vi "CDW_SpecPage.vi"(10 "Spec Page Interface":T2, 11 "MetaDataObj in":refnum<class "MetaDataObj.lvclass">) -> (3 "MetaDataObj out":refnum<class "MetaDataObj.lvclass">)   [LabVIEW 2015, in "NIVS_CDW_MetaDataObj.lvclass"]
uses:
  NIVS_CDW_MetaDataObj.lvclass
  <resource>/dialog/NewProjectWizard/Spec Page Interface.ctl
  <resource>/dialog/NewProjectWizard/MetaDataObj/MetaDataObj.lvclass
  <vilib>/Utility/sysdir.llb/System Directory Type.ctl
  TypDef/CD Wizard - Execution Mode.ctl
  NIVS_CDW_MetaDataObj.lvclass/NIVS_CDW_MetaDataObj.ctl
  <resource>/dialog/NewProjectWizard/MetaDataObj/MetaDataObj.lvclass/MetaDataObj.ctl
  TypDef/CD Wizard - Extra Page Name and GUID.ctl
  <resource>/dialog/NewProjectWizard/MetaDataObj/Accessors/Write Project Root.vi
  <resource>/dialog/NewProjectWizard/MetaDataObj/Accessors/Write Project Name.vi
panel:
  in  "Custom Device Execution Mode":T1(ring)=enum."Inline HW Interface"
  in  "Custom Device Name":string
  in  "Custom Device Path":path
  in  "Maximum Custom Device Instances":u32=1 min=1 max=2474 step=1
  in  "Insert Custom Device in submenu":bool
  in  "Parent Menu Name":string
  in  "Custom Device Extra Page Names":string[](array[string])
  # "Advanced Options"
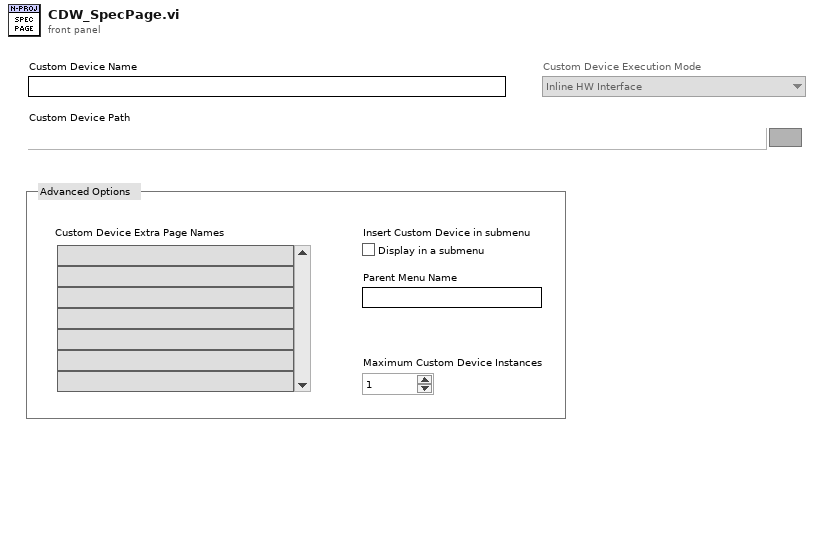
[diagram p1: front panel]
types:
  T1 = enum16{"Asynchronous", "Inline HW Interface", "Inline Model Interface", "Inline Timing and Sync", "Asynchronous Timing and Sync"}
  T2 = typedef "Spec Page Interface.ctl" = cluster{"\"Tab Forward To\" Refnum":refnum<vi>, "\"Tab Backward To\" Refnum":refnum<vi>, "Errors":refnum<user-event>, "Quit":refnum<user-event>}
  T3 = typedef "CD Wizard - Execution Mode.ctl" = enum16{"Asynchronous", "Inline HW Interface", "Inline Model Interface", "Inline Timing and Sync", "Asynchronous Timing and Sync"}
  T4 = typedef "System Directory Type.ctl" = i32
  T5 = enum8{"Enabled", "Disabled", "Disabled and Grayed Out"}
  T6 = cluster{"Insert CD in submenu":bool, "Parent Menu Name":string}
  T7 = typedef "CD Wizard - Extra Page Name and GUID.ctl" = cluster{"Page Name":string, "Page GUID":string}
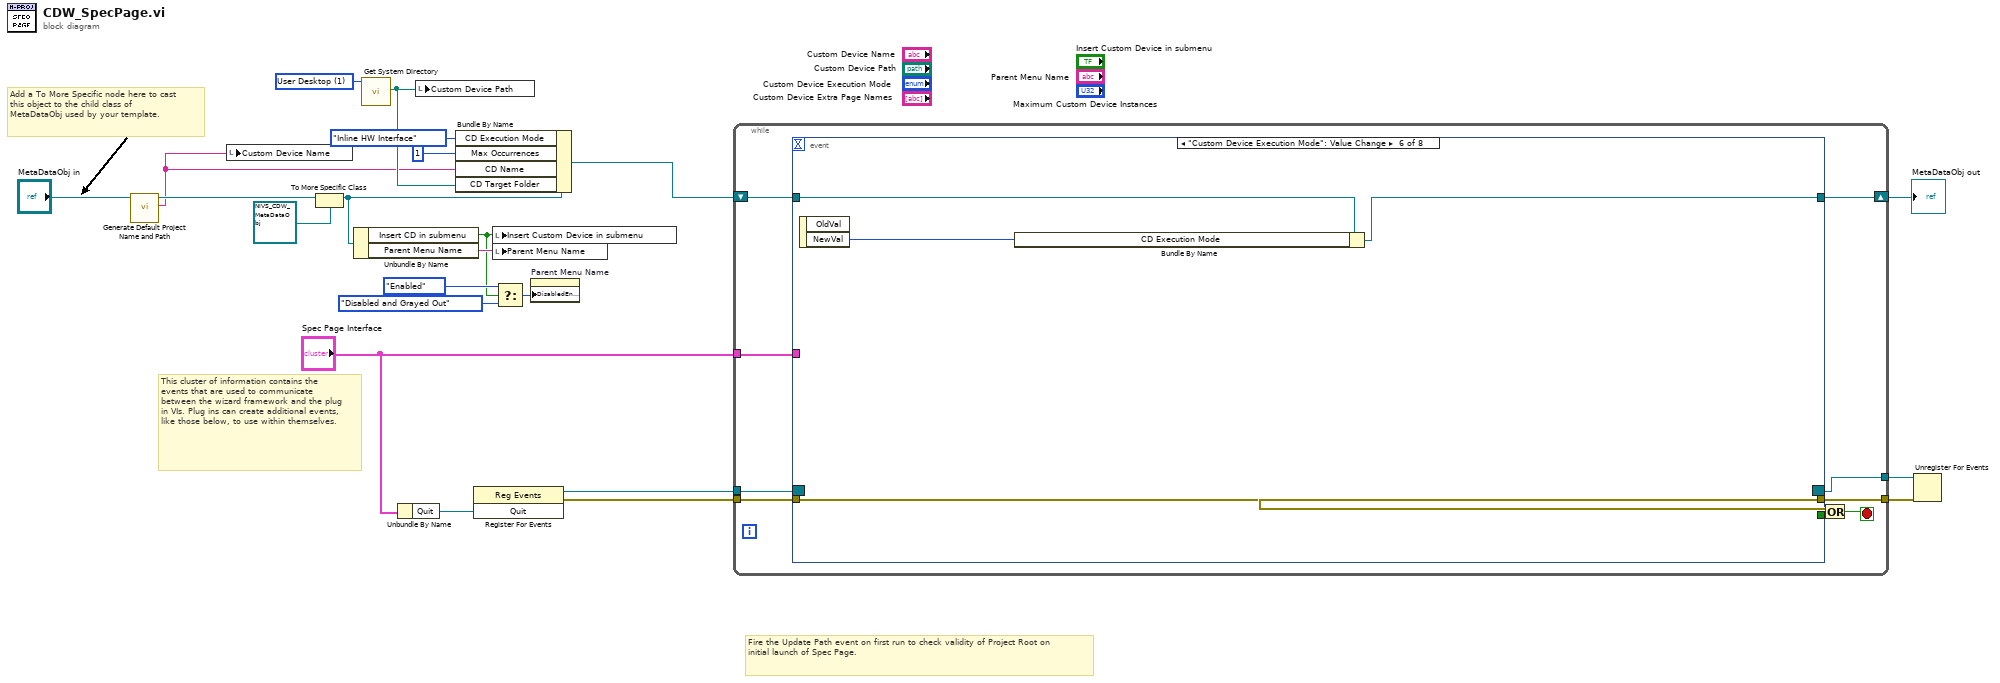
[diagram p0: block diagram]
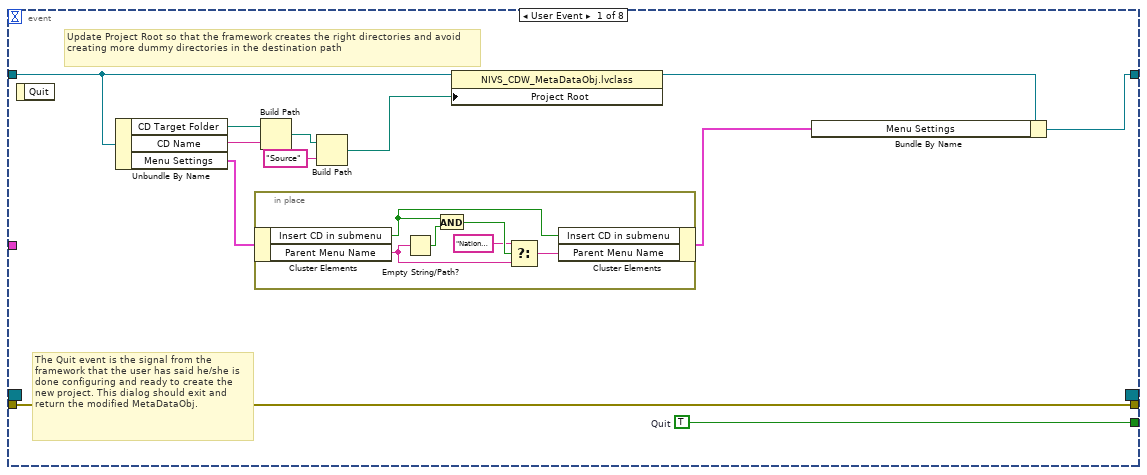
[diagram p2: hidden frame]
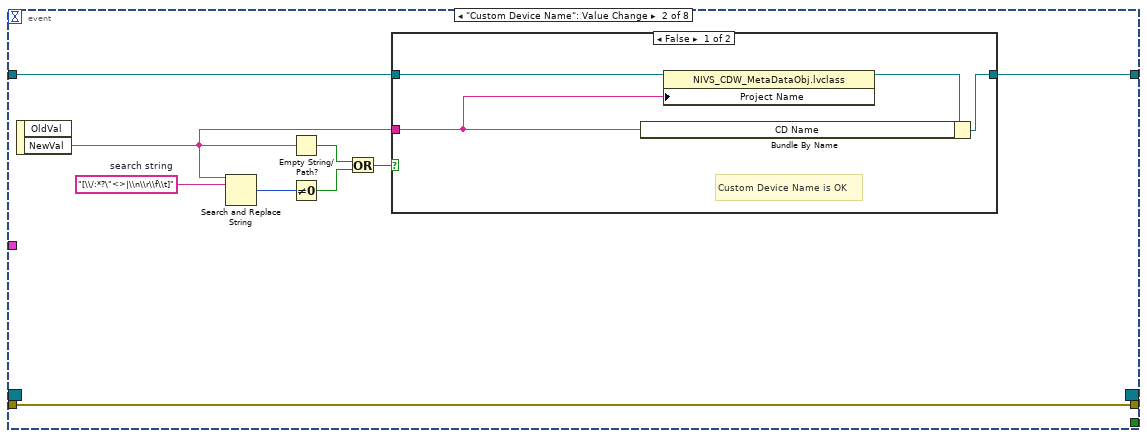
[diagram p3: hidden frame]
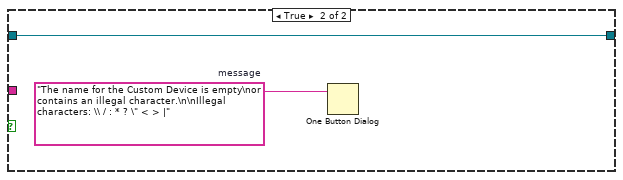
[diagram p4: hidden frame]
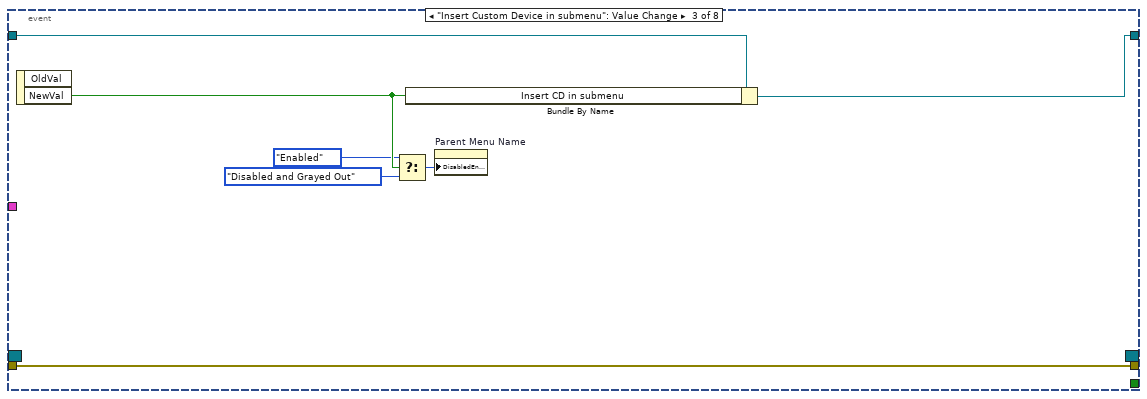
[diagram p5: hidden frame]
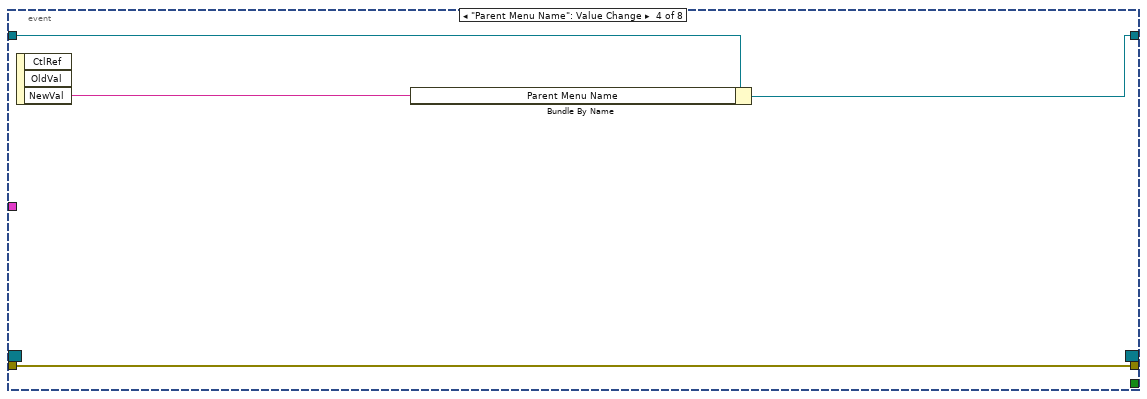
[diagram p6: hidden frame]
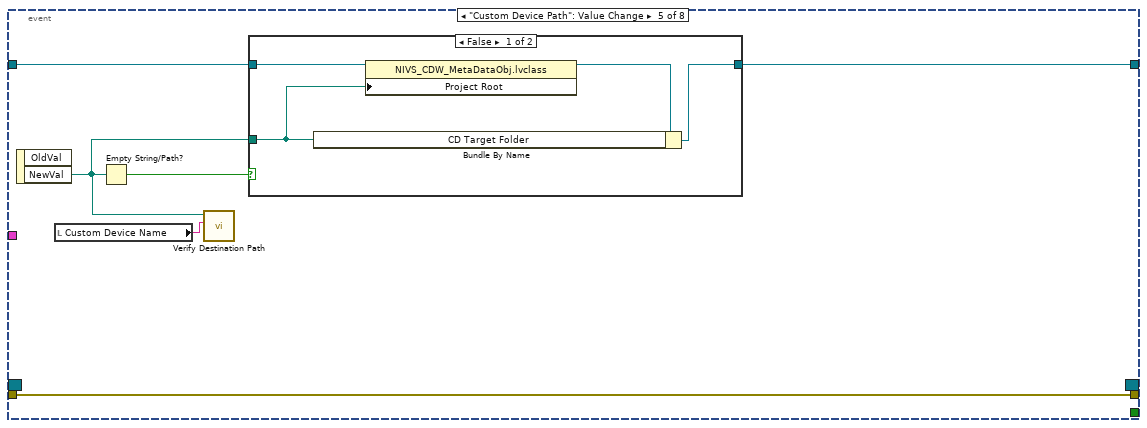
[diagram p7: hidden frame]
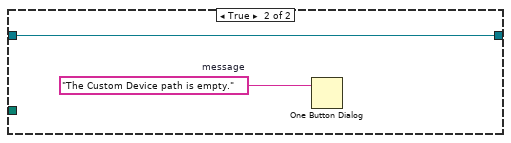
[diagram p8: hidden frame]
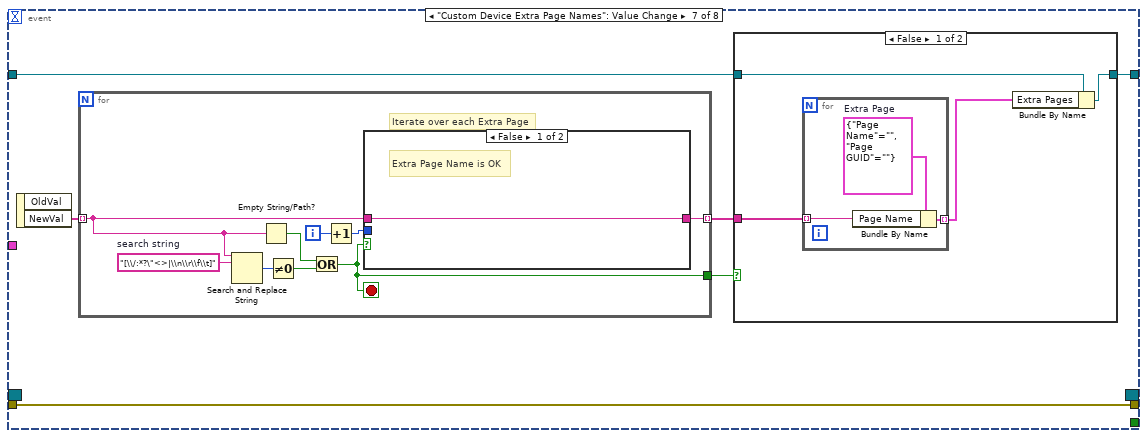
[diagram p9: hidden frame]
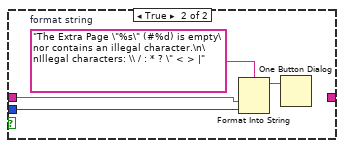
[diagram p11: hidden frame]
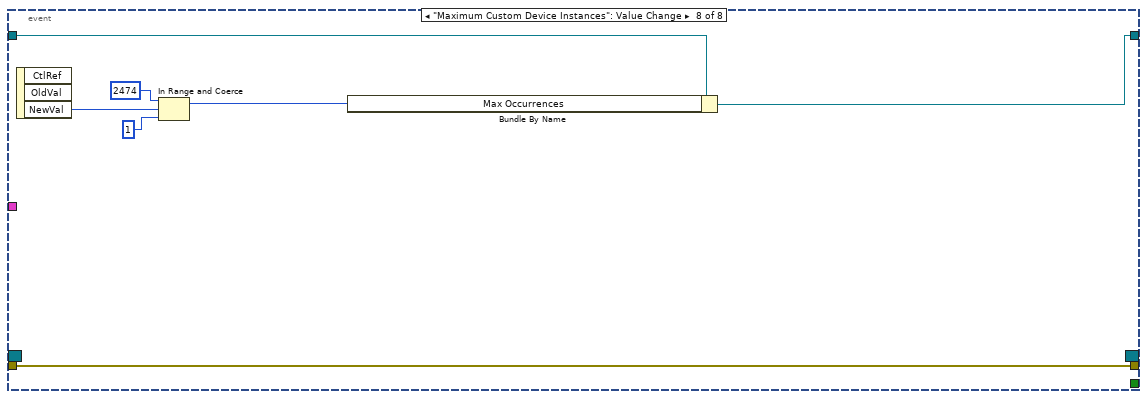
[diagram p12: hidden frame]
diagram:
  w8 = T4 1 items=["User Home"=0, "User Desktop"=1, "User Documents"=2, "User Application Data"=3, "User Preferences"=4, "User Temporary"=5, "Public Documents"=6, "Public Application Data"=7, "Public Preferences"=8, "Public Cache"=13, "System Core Libraries"=9, "System Installed Libraries"=10, "Application Files"=11, "Boot Volume Root"=12] ("system directory type")
  # "Fire the Update Path event on first run to check validity of Project Root on initial launch of Spec Page."
  # "This cluster of information contains the events that are used to communicate between the wizard framework and the plug in VIs. Plug ins can create additional events, like those below, to use within themselves."
  # "Add a To More Specific node here to cast this object to the child class of MetaDataObj used by your template."
  n1 = call <resource>:"Generate Default Project Name and Path.vi"("DNL_MetaDataObj in"="MetaDataObj in") -> ("Project Name"=w5:string, "DNL_MetaDataObj out"=w15:refnum<class "MetaDataObj.lvclass">)  [unwired: 8 in, 1 out]
  n2 = local write "Custom Device Name"(w5) -> ()
  n3 = To More Specific Class(target class=refnum<class "NIVS_CDW_MetaDataObj.lvclass"> refnum ("NIVS_CDW_MetaDataObj.lvclass"), reference=w15) -> (specific class reference=w7:refnum<class "NIVS_CDW_MetaDataObj.lvclass">)  [unwired: 1 in, 1 out]
  n4 = Unbundle By Name(w7) -> ("Insert CD in submenu"=w9:bool, "Parent Menu Name"=w13:string)
  n5 = call <vilib>:"Get System Directory.vi"("system directory type"=w8) -> ("system directory"=w6:path)  [unwired: 10 in]
  n6 = Unbundle By Name("Spec Page Interface") -> ("Quit"=w22:refnum<user-event>)
  n7 = local write "Custom Device Path"(w6) -> ()
  n8 = Bundle By Name(cluster=w7, "CD Execution Mode"=CD_Wizard_-_Execution_Mode."Inline HW Interface" ("CD Wizard - Internal Data.Common Information.CD Execution Mode"), "Max Occurrences"=u32 1 ("CD Wizard - Internal Data.Common Information.Max Occurrences"), "CD Name"=w5, "CD Target Folder"=w6) -> (w4:refnum<class "NIVS_CDW_MetaDataObj.lvclass">)
  n9 = register-events(w22) -> (reference out=w21:refnum<event-registration>, error out=w16:errorcluster)  [unwired: 2 in]
  n10 = local write "Insert Custom Device in submenu"(w9) -> ()
  n11 = local write "Parent Menu Name"(w13) -> ()
  n12 = Select(t=T5."Enabled" ("Disabled"), s=w9, f=T5."Disabled and Grayed Out") -> (s? t:f=w12:T5)
  n13 = property on="Parent Menu Name" class="Str"("DisabledEnum"=w12) -> ()  [unwired: 2 in, 2 out]
  n14 = while {
    tunnel: "Spec Page Interface" -> [w29]
    shift-right: [w28] -> w18
    shift-left: w4 -> [w27]
    tunnel: w21 -> [w31]
    tunnel: w16 -> [w30]
    tunnel: [w24] -> w19
    tunnel: [w23] -> w2
    stop <- w26 stop-if-true
    n15 = event shown="[5] \"Custom Device Execution Mode\": Value Change" {
      selector: w31 -> [_ _ _ _ _ _ _ _]
      dyn-events: [_ _ _ _ _ _ _ _] -> w23
      timeout: _ -> [_ _ _ _ _ _ _ _]
      tunnel: w29 -> [_ _ _ _ _ _ _ _]
      tunnel: [w43 _ _ _ _ _ _ _] -> w25
      tunnel: [w42 w58 w71 w75 w81 w91 w97 w126] -> w24
      tunnel: w30 -> [w42 w58 w71 w75 w81 w91 w97 w126]
      tunnel: [w34 w52 w69 w73 w78 w89 w93 w124] -> w28
      tunnel: w27 -> [w41 w50 w70 w74 w79 w90 w94 w125]
      event User Event {
        w43 = TRUE  # Quit
        # "Update Project Root so that the framework creates the right directories and avoid creating more dummy directories in the destination path"
        # "The Quit event is the signal from the framework that the user has said he/she is done configuring and ready to create the new project. This dialog should exit and return the modified MetaDataObj."
        n16 = event-data() -> ()  [unwired: 1 in, 1 out]
        n17 = Unbundle By Name(w41) -> ("CD Target Folder"=w40:path, "CD Name"=w36:string, "Menu Settings"=w33:T6)
        n18 = in-place {
          n19 = in-place-cluster #1(w33) -> ("Insert CD in submenu"=w45:bool, "Parent Menu Name"=w48:string)
          n20 = Empty String/Path?(string/path=w48) -> (empty?=w49:bool)
          n21 = And(x=w45, y=w49) -> (x .and. y?=w46:bool)
          n22 = Select(t="National Instruments", s=w46, f=w48) -> (s? t:f=w47:string)
          n23 = in-place-cluster #1("Insert CD in submenu"=w45, "Parent Menu Name"=w47) -> (w32:T6)
        }
        n24 = Build Path(base path=w40, name or relative path=w36) -> (appended path=w39:path)
        n25 = Build Path(base path=w39, name or relative path="Source") -> (appended path=w37:path)
        n26 = property class="NIVS_CDW_MetaDataObj.lvclass"(reference=w41, "Project Root"=w37) -> (reference out=w35:refnum<class "NIVS_CDW_MetaDataObj.lvclass">)  [unwired: 1 in, 1 out]
        n27 = Bundle By Name(cluster=w35, "Menu Settings"=w32) -> (w34:refnum<class "NIVS_CDW_MetaDataObj.lvclass">)
      }
      event "Custom Device Name": Value Change {
        w54 = "[\\/:*?\"<>|\\n\\r\\f\\t]"  # search string
        n28 = event-data() -> ("NewVal"=w51:string)  [unwired: 1 in, 1 out]
        n29 = Search and Replace String(input string=w51, search string=w54) -> (number of replacements=w55:i32)  [unwired: 6 in, 3 out]
        n30 = Empty String/Path?(string/path=w51) -> (empty?=w56:bool)
        n31 = Not Equal To 0?(x=w55) -> (x != 0?=w57:bool)
        n32 = Or(x=w56, y=w57) -> (x .or. y?=w53:bool)
        n33 = case shown="False" w53 {
          tunnel: w50 -> [w61 w63]
          tunnel: [w62 w63] -> w52
          tunnel: w51 -> [w59 _]
          frame False {
            # "Custom Device Name is OK"
            n34 = property class="NIVS_CDW_MetaDataObj.lvclass"(reference=w61, "Project Name"=w59) -> (reference out=w60:refnum<class "NIVS_CDW_MetaDataObj.lvclass">)  [unwired: 1 in, 1 out]
            n35 = Bundle By Name(cluster=w60, "CD Name"=w59) -> (w62:refnum<class "NIVS_CDW_MetaDataObj.lvclass">)
          }
          frame True {
            w64 = "The name for the Custom Device is empty\nor contains an illegal character.\n\nIllegal characters: \\ / : * ? \" < > |"  # message
            n36 = One Button Dialog(message=w64) -> ()  [unwired: 1 in, 1 out]
          }
        }
      }
      event "Insert Custom Device in submenu": Value Change {
        n37 = event-data() -> ("NewVal"=w68:bool)  [unwired: 1 in, 1 out]
        n38 = Select(t=T5."Enabled" ("Disabled"), s=w68, f=T5."Disabled and Grayed Out") -> (s? t:f=w65:T5)
        n39 = Bundle By Name(cluster=w70, "Insert CD in submenu"=w68) -> (w69:refnum<class "NIVS_CDW_MetaDataObj.lvclass">)
        n40 = property on="Parent Menu Name" class="Str"("DisabledEnum"=w65) -> ()  [unwired: 2 in, 2 out]
      }
      event "Parent Menu Name": Value Change {
        n41 = event-data() -> ("NewVal"=w72:string)  [unwired: 1 in, 2 out]
        n42 = Bundle By Name(cluster=w74, "Parent Menu Name"=w72) -> (w73:refnum<class "NIVS_CDW_MetaDataObj.lvclass">)
      }
      event "Custom Device Path": Value Change {
        n43 = event-data() -> ("NewVal"=w77:path)  [unwired: 1 in, 1 out]
        n44 = local read "Custom Device Name"() -> (w76:string)
        n45 = Empty String/Path?(string/path=w77) -> (empty?=w80:bool)
        n46 = call "Verify Destination Path.vi"("Custom Device Name"=w76, "Custom Device Path"=w77) -> ()  [unwired: 9 in, 1 out]
        n47 = case shown="False" w80 {
          tunnel: w79 -> [w84 w86]
          tunnel: [w85 w86] -> w78
          tunnel: w77 -> [w82 _]
          frame False {
            n48 = property class="NIVS_CDW_MetaDataObj.lvclass"(reference=w84, "Project Root"=w82) -> (reference out=w83:refnum<class "NIVS_CDW_MetaDataObj.lvclass">)  [unwired: 1 in, 1 out]
            n49 = Bundle By Name(cluster=w83, "CD Target Folder"=w82) -> (w85:refnum<class "NIVS_CDW_MetaDataObj.lvclass">)
          }
          frame True {
            w87 = "The Custom Device path is empty."  # message
            n50 = One Button Dialog(message=w87) -> ()  [unwired: 1 in, 1 out]
          }
        }
      }
      event "Custom Device Execution Mode": Value Change {
        n51 = event-data() -> ("NewVal"=w88:T1)  [unwired: 1 in, 1 out]
        n52 = Bundle By Name(cluster=w90, "CD Execution Mode"=w88) -> (w89:refnum<class "NIVS_CDW_MetaDataObj.lvclass">)
      }
      event "Custom Device Extra Page Names": Value Change {
        n53 = event-data() -> ("NewVal"=w96:string[])  [unwired: 1 in, 1 out]
        n54 = for {
          tunnel: w96 -> [w108] mode=indexing
          tunnel: [w107] -> w95
          tunnel: [w106] -> w92 mode=indexing
          i -> [w110]
          stop <- w107 stop-if-true
          w114 = "[\\/:*?\"<>|\\n\\r\\f\\t]"  # search string
          # "Iterate over each Extra Page"
          n55 = Search and Replace String(input string=w108, search string=w114) -> (number of replacements=w113:i32)  [unwired: 6 in, 3 out]
          n56 = Empty String/Path?(string/path=w108) -> (empty?=w112:bool)
          n57 = Not Equal To 0?(x=w113) -> (x != 0?=w111:bool)
          n58 = Or(x=w112, y=w111) -> (x .or. y?=w107:bool)
          n59 = Increment(x=w110) -> (x+1=w109:i32)
          n60 = case shown="False" w107 {
            tunnel: w109 -> [_ w116]
            tunnel: w108 -> [w115 w117]
            tunnel: [w115 _] -> w106
            frame False {
              # "Extra Page Name is OK"
            }
            frame True {
              w119 = "The Extra Page \"%s\" (#%d) is empty\nor contains an illegal character.\n\nIllegal characters: \\ / : * ? \" < > |"  # format string
              n61 = Format Into String(format string=w119, w117, w116) -> (resulting string=w118:string)  [unwired: 2 in, 1 out]
              n62 = One Button Dialog(message=w118) -> ()  [unwired: 1 in, 1 out]
            }
          }
        }
        n63 = case shown="False" w95 {
          tunnel: w94 -> [w101 w105]
          tunnel: [w100 w105] -> w93
          tunnel: w92 -> [w98 _]
          frame False {
            n64 = for {
              tunnel: [w103] -> w99 mode=indexing
              tunnel: w98 -> [w102] mode=indexing
              w104 = T7 {"Page Name"="", "Page GUID"=""}  # Extra Page
              n65 = Bundle By Name(cluster=w104, "Page Name"=w102) -> (w103:T7)
            }
            n66 = Bundle By Name(cluster=w101, "Extra Pages"=w99) -> (w100:refnum<class "NIVS_CDW_MetaDataObj.lvclass">)
          }
          frame True {
          }
        }
      }
      event "Maximum Custom Device Instances": Value Change {
        n67 = event-data() -> ("NewVal"=w123:u32)  [unwired: 1 in, 2 out]
        n68 = In Range and Coerce(upper limit=u32 2474, x=w123, lower limit=u32 1) -> (coerced(x)=w120:u32)  [unwired: 1 out]
        n69 = Bundle By Name(cluster=w125, "Max Occurrences"=w120) -> (w124:refnum<class "NIVS_CDW_MetaDataObj.lvclass">)
      }
    }
    n70 = Or(x=w24, y=w25) -> (x .or. y?=w26:bool)
  }
  "MetaDataObj out" <- w18
  n71 = Unregister For Events(event registration refnum=w2, error in=w19) -> ()  [unwired: 1 out]
